vi "Arduino_Unfinished_Read from SD and Drive LEDs.vi"() -> ()   [LabVIEW 2015]
doc: "This example demonstrates a rainbow effect on a 1-wire RGB LED strip using a WS2811 or WS2812 controller. Each LED in the strip is gradually changed from red to green, then to blue with a blend of colors in between. The LED color changing effect is staggered down the strip so not all LEDs are changed at the same time. The time delay can also be adjusted to change how fast the color is changed."
uses:
  <vilib>/Aledyne-TSXperts/Arduino Compatible Compiler for LabVIEW/Code Generator/Arduino APIs/RGB LED Strip/RGB Strip Mode.ctl
  <vilib>/Aledyne-TSXperts/Arduino Compatible Compiler for LabVIEW/Arduino Compatible Compiler for LabVIEW.lvlib
panel:
  in  "Mode":T1=3 items=["400kHz_RGB"=0, "400kHz_GRB"=1, "400kHz_BRG"=4, "800kHz_RGB"=2, "800kHz_GRB"=3, "400kHz_BRG"=6]
  in  "Digital Pin":u8=4
  # "Overview: Demonstrates a rainbow effect on a 1-wire RGB LED strip using a WS2811 or WS2812 controller.  Each LED in the strip is gradually changed from red to green, then to blue with a blend of colors in between.  The LED color changing effect is staggered down the strip so not all LEDs are changed at the same time.  The time delay can also be adjusted to change how fast the color is changed.\n\nInstructions:\n1. Wire a 1-wire LED strip to a digital pin on the Arduino board.  Follow wiring instructions from the manufacturer.  A 100-500 ohm resistor is usually recommended between the Arduino digital output and the LED strip's data in pin.  Also, a 100 uF capacitor between the ground and power input may reduce noise on from the power supply.  It is also recommended to power the LED strip from a separate power input if available on the strip.  When daisy chaining LED strips, it is recommended to only daisy chain the Data line and to power each strip from a separate power input.\n2. Set the Digital Pin wired below.\n3. Set the Mode to the correct setting for your LED strip (the WS2812 uses 800kHz GRB).\n4. Set the Number of LEDs on your strip.  This can be set to any number equal to or smaller than the number of physical LEDs on the strip of you do not wish to power up all of them.\n5. Set the delay (ms) between changes to the LED color.\n6.  If this example has been loaded from the Arduino Compatible Compiler for LabVIEW, simply select Compile and Download.  Otherwise, open Tools>Arduino Compatible Compiler for LabVIEW in LabVIEW, then select File>Load VI, and select this VI and then Compile and Download.\n7. Observe the LEDs on the strip changing color with a seamless rainbow transition."
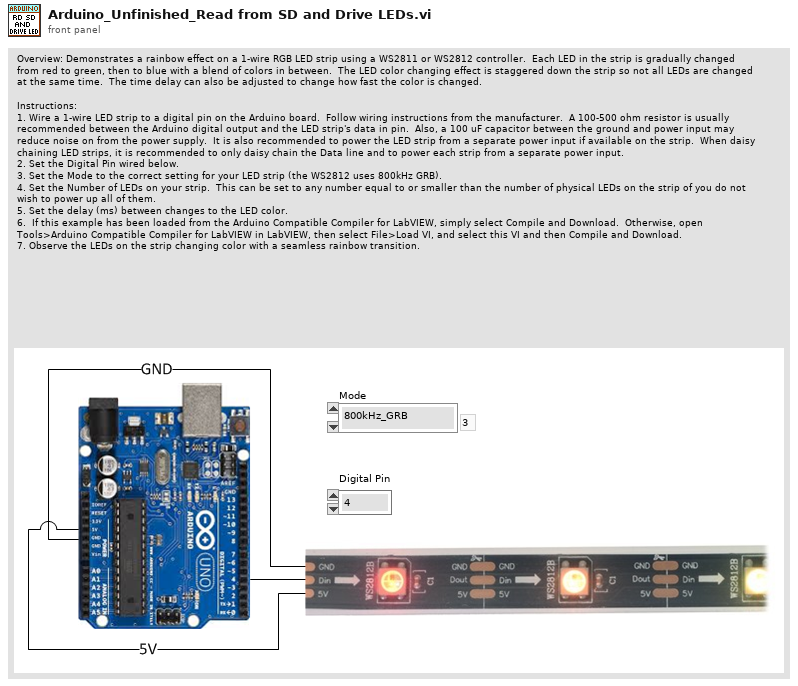
[diagram p1: front panel]
types:
  T1 = typedef "Arduino Compatible Compiler for LabVIEW.lvlib/RGB Strip Mode.ctl" = u16
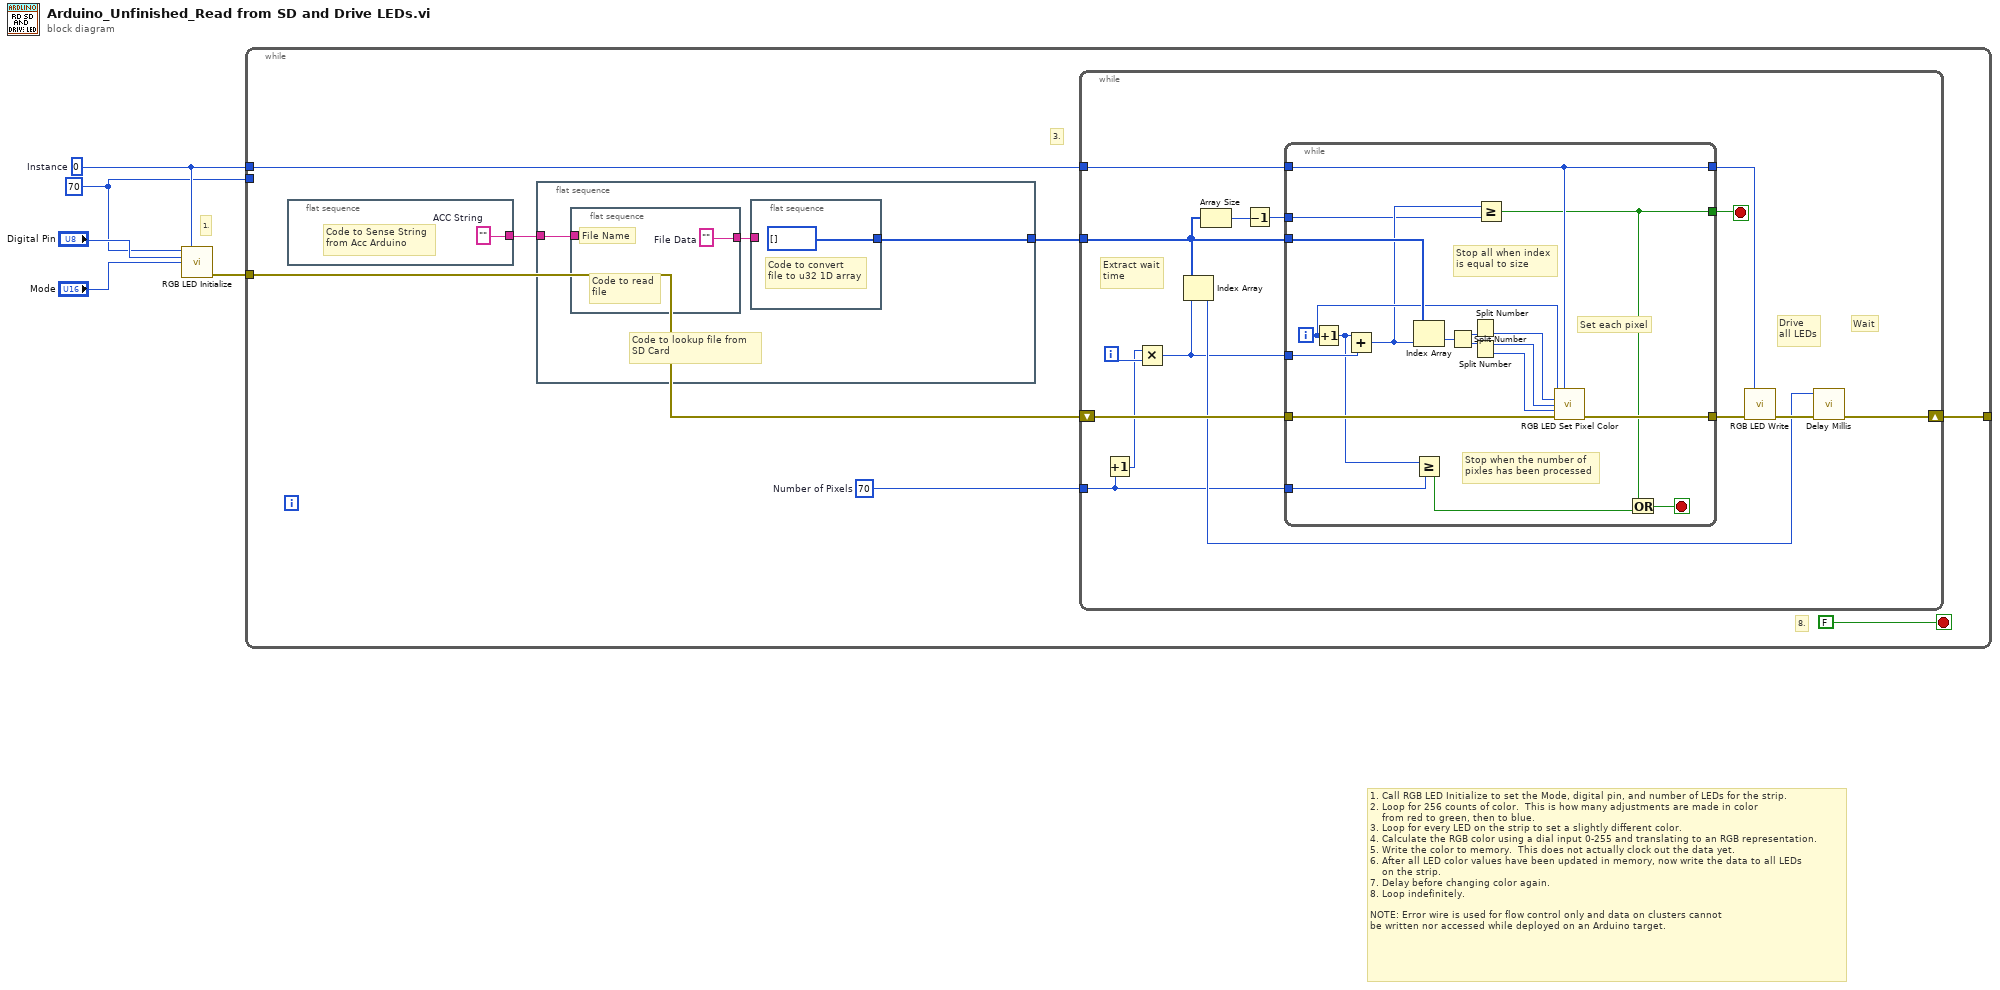
[diagram p0: block diagram]
diagram:
  w1 = u16 70 ("Number of LEDs")
  w2 = u8 0  # Instance
  # "1."
  # "1. Call RGB LED Initialize to set the Mode, digital pin, and number of LEDs for the strip.\n2. Loop for 256 counts of color.  This is how many adjustments are made in color\n    from red to green, then to blue.\n3. Loop for every LED on the strip to set a slightly different color.\n4. Calculate the RGB color using a dial input 0-255 and translating to an RGB representation.\n5. Write the color to memory.  This does not actually clock out the data yet.\n6. After all LED color values have been updated in memory, now write the data to all LEDs\n    on the strip.\n7. Delay before changing color again.\n8. Loop indefinitely.\n\nNOTE: Error wire is used for flow control only and data on clusters cannot\nbe written nor accessed while deployed on an Arduino target."
  n1 = call <vilib>:"RGB LED Initialize.vi"("Number of Pixels"=w1, "Instance"=w2, "Pin"="Digital Pin", "Mode"="Mode") -> ("error out"=w3:errorcluster)  [unwired: 11 in]
  n2 = while {
    tunnel: w3 -> [w11]
    tunnel: w2 -> [w10]
    tunnel: w1 -> [_]
    tunnel: [w9] -> _
    stop <- FALSE stop-if-true
    w6 = 70  # Number of Pixels
    # "3."
    # "8."
    n3 = flat-sequence {
      tunnel: [w52] -> w8
      frame #0 {
        w52 = ""  # ACC String
        # "Code to Sense String\nfrom Acc Arduino"
      }
    }
    n4 = flat-sequence {
      tunnel: w8 -> [w49]
      tunnel: [w47] -> w7
      frame #0 {
        # "Code to lookup file from\nSD Card"
        n5 = flat-sequence {
          tunnel: w49 -> [_]
          tunnel: [w51] -> w48
          frame #0 {
            w51 = ""  # File Data
            # "File Name"
            # "Code to read\nfile"
          }
        }
        n6 = flat-sequence {
          tunnel: w48 -> [_]
          tunnel: [u32[] []] -> w47
          frame #0 {
            # "Code to convert\nfile to u32 1D array"
          }
        }
      }
    }
    n7 = while {
      tunnel: w10 -> [w26]
      tunnel: w7 -> [w18]
      shift-right: [w25] -> w9
      shift-left: w11 -> [w27]
      tunnel: w6 -> [w19]
      i -> [w17]
      stop <- w13 stop-if-true
      # "Extract wait\ntime"
      # "Wait"
      # "Drive\nall LEDs"
      n8 = Increment(x=w19) -> (x+1=w15:i32)
      n9 = Multiply(x=w15, y=w17) -> (x*y=w20:i32)
      n10 = Index Array(array=w18, index=w20) -> (element=w21:u32)
      n11 = Array Size(array=w18) -> (size(s)=w16:i32)
      n12 = Decrement(x=w16) -> (x-1=w14:i32)
      n13 = while {
        tunnel: w26 -> [w44]
        tunnel: w27 -> [w46]
        tunnel: [w45] -> w23
        tunnel: [w44] -> w22
        tunnel: w18 -> [w39]
        tunnel: w20 -> [w43]
        tunnel: w19 -> [w41]
        tunnel: w14 -> [w29]
        tunnel: [w28] -> w13
        i -> [w32]
        stop <- w31 stop-if-true
        # "Set each pixel"
        # "Stop all when index\nis equal to size"
        # "Stop when the number of\npixles has been processed"
        n14 = Increment(x=w32) -> (x+1=w42:i32)
        n15 = Add(x=w42, y=w43) -> (x+y=w30:i32)
        n16 = Index Array(array=w39, index=w30) -> (element=w38:u32)
        n17 = Greater Or Equal?(x=w42, y=w41) -> (x >= y?=w40:bool)
        n18 = Split Number(x=w38) -> (hi(x)=w37:u16, lo(x)=w36:u16)
        n19 = Split Number(x=w37) -> (lo(x)=w35:u8)  [unwired: 1 out]
        n20 = Split Number(x=w36) -> (hi(x)=w34:u8, lo(x)=w33:u8)
        n21 = Greater Or Equal?(x=w30, y=w29) -> (x >= y?=w28:bool)
        n22 = call <vilib>:"RGB LED Set Pixel Color.vi"("Pixel"=w32, "Instance"=w44, "Red"=w35, "Green"=w34, "Blue"=w33, "error in (no error)"=w46) -> ("error out"=w45:errorcluster)  [unwired: 9 in]
        n23 = Or(x=w28, y=w40) -> (x .or. y?=w31:bool)
      }
      n24 = call <vilib>:"RGB LED Write.vi"("Instance"=w22, "error in (no error)"=w23) -> ("error out"=w24:errorcluster)  [unwired: 13 in]
      n25 = call <vilib>:"Delay Millis.vi"("error in (no error)"=w24, "delay"=w21) -> ("error out"=w25:errorcluster)  [unwired: 9 in]
    }
  }
